vi "Stiffness (SubVI).vi"(0 "C_DBP":dbl, 1 "C_SBP":dbl, 2 "dD":dbl, 3 "Dd":dbl) -> (7 "Beta":dbl, 8 "Ep":dbl, 9 "AC":dbl, 10 "PWV_b":dbl)   [LabVIEW 2017]
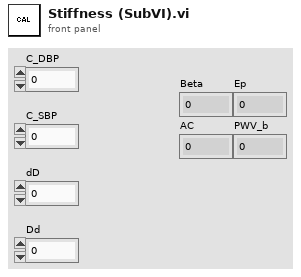
[diagram p1: front panel]
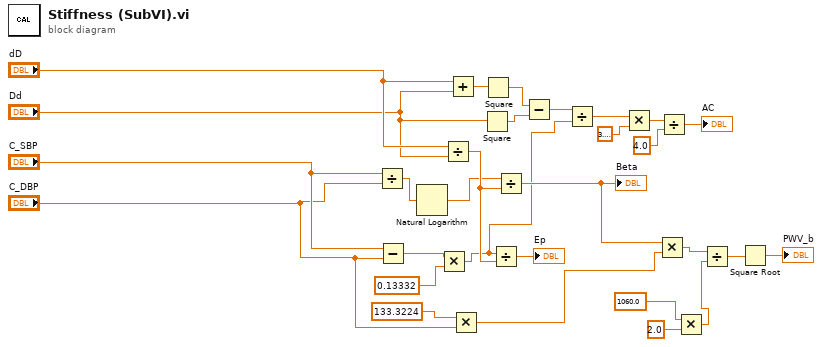
[diagram p0: block diagram]
diagram:
  n1 = Divide(x="C_SBP", y="C_DBP") -> (x/y=w8:dbl)
  n2 = Subtract(x="C_SBP", y="C_DBP") -> (x-y=w5:dbl)
  n3 = Natural Logarithm(1:w8) -> (0:w7:dbl)
  n4 = Multiply(x=w5, y=0.13332) -> (x*y=w4:dbl)
  n5 = Divide(x="dD", y="Dd") -> (x/y=w28:dbl)
  n6 = Add(x="dD", y="Dd") -> (x+y=w25:dbl)
  n7 = Multiply(x=133.3224 ("y"), y="C_DBP") -> (x*y=w1:dbl)
  n8 = Square(x="Dd") -> (x^2=w22:dbl)
  n9 = Square(x=w25) -> (x^2=w23:dbl)
  n10 = Divide(x=w4, y=w28) -> (x/y=→"Ep":dbl)
  n11 = Divide(x=w7, y=w28) -> (x/y=w9:dbl)
  "Beta" <- w9
  n12 = Subtract(x=w23, y=w22) -> (x-y=w21:dbl)
  n13 = Divide(x=w21, y=w4) -> (x/y=w20:dbl)
  n14 = Multiply(x=w20, y=3.141592653589793) -> (x*y=w18:dbl)
  n15 = Multiply(x=w9, y=w1) -> (x*y=w15:dbl)
  n16 = Divide(x=w18, y=4.0) -> (x/y=→"AC":dbl)
  n17 = Multiply(x=1060.0 ("y"), y=2.0) -> (x*y=w12:dbl)
  n18 = Divide(x=w15, y=w12) -> (x/y=w11:dbl)
  n19 = Square Root(x=w11) -> (sqrt(x)=→"PWV_b":dbl)
